vi "Identity Value.vi"(3 "DataProc Identity in":refnum<class "DataProc Identity.lvclass">) -> (1 "Value":string)   [LabVIEW 2020, in "VolatusData.lvlib" / "DataProc Identity.lvclass"]
uses:
  DataProc Identity.lvclass
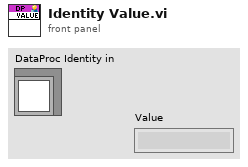
[diagram p1: front panel]
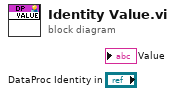
[diagram p0: block diagram]
diagram:
